vi "GenerateSTP_Tx Payload.vi"(8 "error in (no error)":errorcluster, 11 "STP Protocol in":refnum<class "STP Protocol.lvclass">) -> (0 "error out":errorcluster, 3 "STP Protocol out":refnum<class "STP Protocol.lvclass">)   [LabVIEW 2023, in "HardwareAbstractionLayer_LVOOP.lvlib" / "CAN Application Protocols Lib.lvlib" / "STP Protocol.lvclass"]
uses:
  STP Protocol.lvclass
  STP Protocol.lvclass/STP Protocol.ctl
  Ctrls/TP Frame Type.ctl
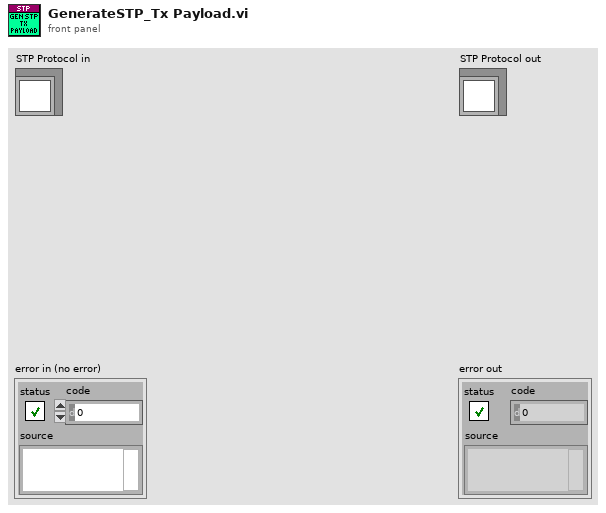
[diagram p1: front panel]
types:
  T1 = typedef "HardwareAbstractionLayer_LVOOP.lvlib/CAN Application Protocols Lib.lvlib/STP Protocol.lvclass/STP CMD.ctl" = u8
  T2 = typedef "HardwareAbstractionLayer_LVOOP.lvlib/CAN Application Protocols Lib.lvlib/STP Protocol.lvclass/TP Frame Type.ctl" = u8
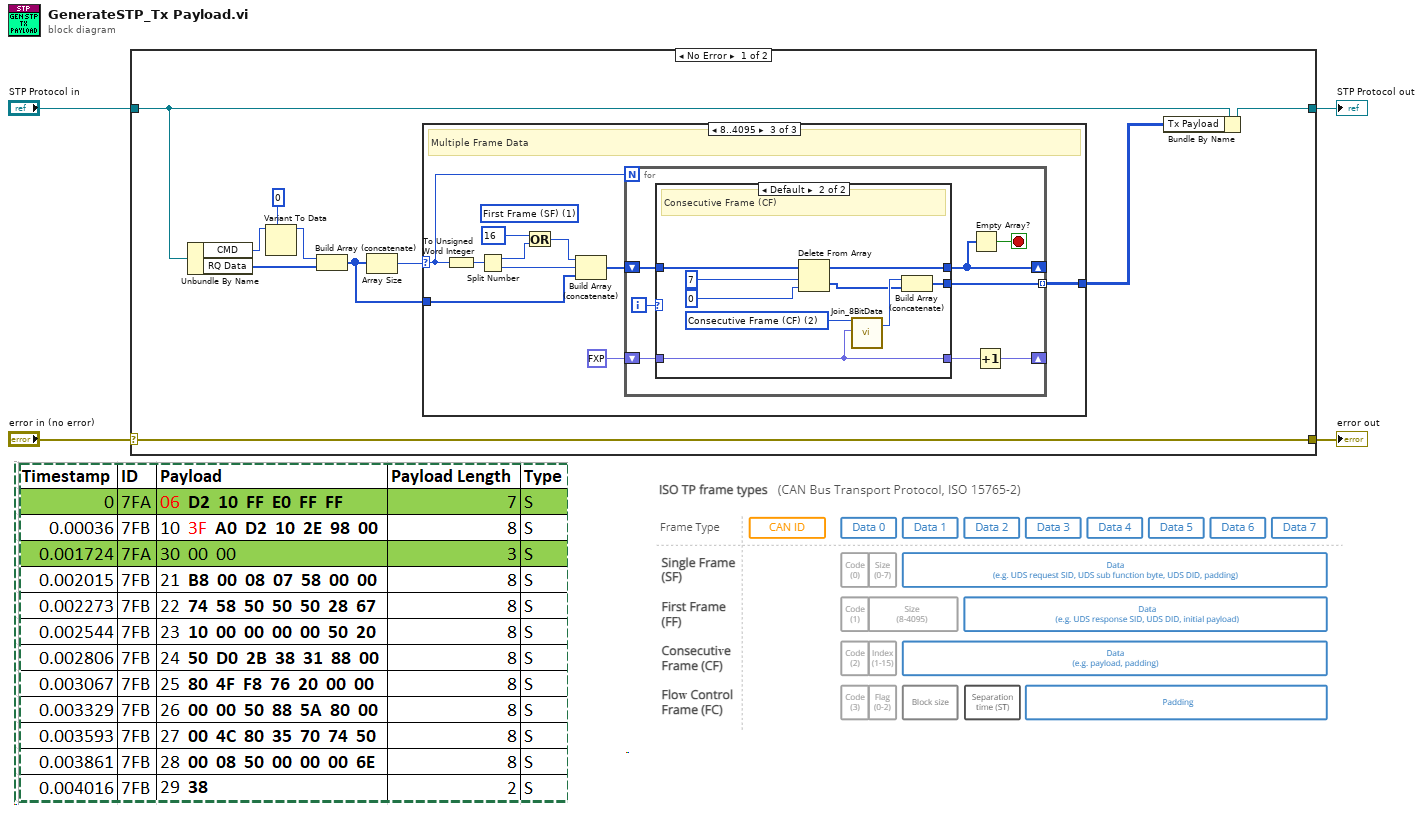
[diagram p0: block diagram]
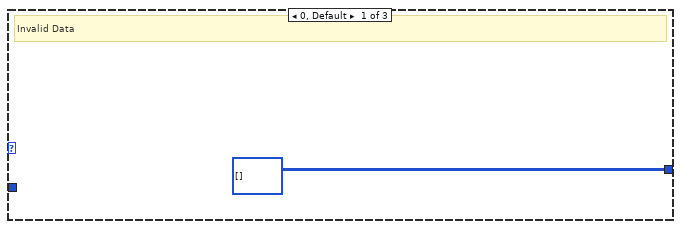
[diagram p2: hidden frame]
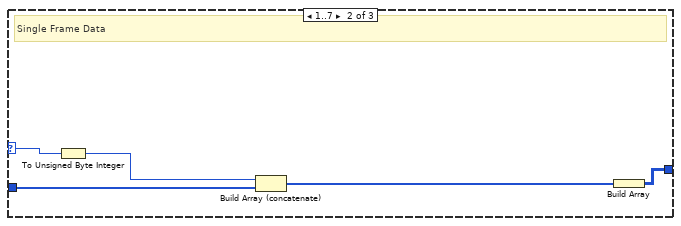
[diagram p3: hidden frame]
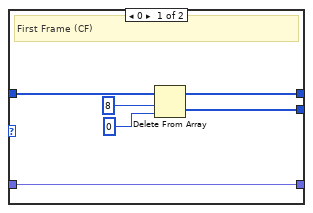
[diagram p4: hidden frame]
diagram:
  n1 = case shown="No Error" "error in (no error)" {
    selector: "error in (no error)" -> [w14 w55]
    tunnel: [w14 w55] -> w3
    tunnel: [w11 w54] -> w1
    tunnel: "STP Protocol in" -> [w13 w54]
    frame No Error {
      n2 = Unbundle By Name(w13) -> ("CMD"=w7:T1, "RQ Data"=w12:u8[])
      n3 = Variant To Data(type=u8 0, Variant=w7) -> (data=w5:u8)  [unwired: 1 in, 1 out]
      n4 = Build Array (concatenate)(w5, w12) -> (w9:u8[])
      n5 = Array Size(array=w9) -> (size(s)=w8:i32)
      n6 = case shown="8..4095" w8 {
        selector: w8 -> [_ w20 w25]
        tunnel: [u8[][] [] ("Tx Payload") w17 w28] -> w10
        tunnel: w9 -> [_ w19 w30]
        frame 0, Default {
          # "Invalid Data"
        }
        frame 1..7 {
          # "Single Frame Data"
          n7 = To Unsigned Byte Integer(number=w20) -> (unsigned 8bit integer=w16:u8)
          n8 = Build Array (concatenate)(w16, w19) -> (w18:u8[])
          n9 = Build Array(w18) -> (w17:u8[][])
        }
        frame 8..4095 {
          (unwired) T2 1 items=["Single Frame (SF)", "First Frame (SF)", "Consecutive Frame (CF)", "Flow Control Frame (FC)"] ("Ring")
          # "Multiple Frame Data"
          n10 = To Unsigned Word Integer(number=w25) -> (unsigned 16bit integer=w24:u16)
          n11 = Split Number(x=w24) -> (hi(x)=w22:u8, lo(x)=w26:u8)
          n12 = Or(x=u8 16, y=w22) -> (x .or. y?=w21:u8)
          n13 = Build Array (concatenate)(w21, w26, w30) -> (w29:u8[])
          n14 = for {
            N: w25 -> [_]
            shift-right: [w31] -> _
            shift-left: w29 -> [w37]
            tunnel: [w36] -> w28 mode=indexing
            shift-right: [w33] -> _
            shift-left: fxp<+,4,4> 0.0 ("CosecutiveFrameID_In") -> [w35]
            i -> [w38]
            stop <- w32 stop-if-true
            n15 = case shown="Default" w38 {
              tunnel: w37 -> [w44 w53]
              tunnel: [w43 w52] -> w31
              tunnel: [w42 w48] -> w36
              tunnel: w35 -> [w39 w49]
              tunnel: [w39 w49] -> w34
              frame 0 {
                # "First Frame (CF)"
                n16 = Delete From Array(array=w44, length=8, index=0) -> (deleted portion=w42:u8[], array with subset deleted=w43:u8[])
              }
              frame Default {
                w45 = T2 2 items=["Single Frame (SF)", "First Frame (SF)", "Consecutive Frame (CF)", "Flow Control Frame (FC)"] ("Ring")
                # "Consecutive Frame (CF)"
                n17 = Delete From Array(array=w53, length=7, index=0) -> (deleted portion=w46:u8[], array with subset deleted=w52:u8[])
                n18 = call "Join_8BitData.vi"("hi"=w45, "lo"=w49) -> ("hi.lo(8bits)"=w47:u8)  [unwired: 17 in]
                n19 = Build Array (concatenate)(w47, w46) -> (w48:u8[])
              }
            }
            n20 = Empty Array?(array=w31) -> (empty?=w32:bool)
            n21 = Increment(x=w34) -> (x+1=w33:fxp<+,4,4>)
          }
        }
      }
      n22 = Bundle By Name(cluster=w13, "Tx Payload"=w10) -> (w11:refnum<class "STP Protocol.lvclass">)
    }
    frame Error {
    }
  }
  "error out" <- w3
  "STP Protocol out" <- w1
